vi "Test Program.vi"() -> ()   [LabVIEW 2018, in "VICI M50.lvlib"]
uses:
  VICI M50/VICI M50.lvlib
  Settings Cluster.ctl
  VICI M6 M50 Party Mode.lvlib
panel:
  out "Connection Error":bool
  out "Pump On?":enum16{"Off", "On", "Not Initialized"}(ring)
  in  "stop":bool
  in  "Pause":bool
  in  "speed":dbl
  out "error in (no error) 2":errorcluster
  in  "error in (no error)":errorcluster
  out "VICI Settings 2":T1={"VISA resource name"="", "Simulated?"=TRUE, "Pump Letter"="", "Reverse?"=FALSE}
  in  "VICI Settings":T1={"VISA resource name"="", "Simulated?"=TRUE, "Pump Letter"="", "Reverse?"=FALSE}
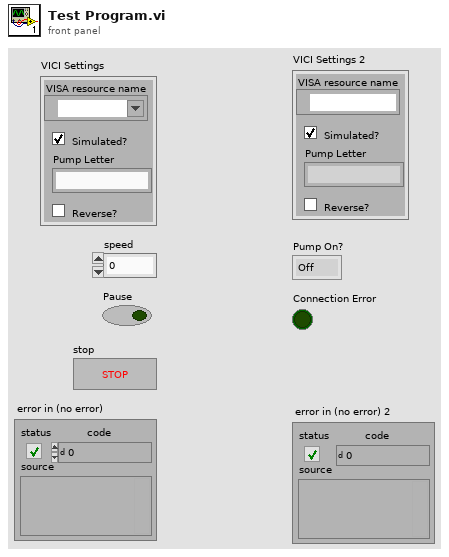
[diagram p1: front panel]
types:
  T1 = typedef "VICI M6 M50 Party Mode.lvlib/Settings Cluster.ctl" = cluster{"VISA resource name":refnum<visa-resource-name>, "Simulated?":bool, "Pump Letter":string, "Reverse?":bool}
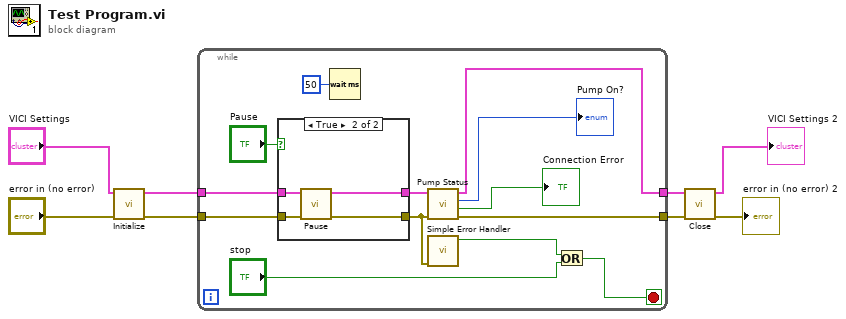
[diagram p0: block diagram]
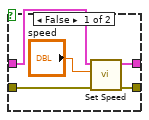
[diagram p2: hidden frame]
diagram:
  n1 = call "Initialize.vi"("error in (no error)"="error in (no error)", "VICI Settings"="VICI Settings") -> ("error out"=w1:errorcluster, "VICI Settings"=w2:T1)  [unwired: 6 in, 2 out]
  n2 = while {
    tunnel: [w21] -> w4
    tunnel: [w20] -> w3
    tunnel: w2 -> [w18]
    tunnel: w1 -> [w17]
    stop <- w13 stop-if-true
    n3 = case shown="True" "Pause" {
      tunnel: [w23 w30] -> w19
      tunnel: [w24 w29] -> w10
      tunnel: w18 -> [w26 w28]
      tunnel: w17 -> [w25 w27]
      frame False {
        n4 = call "Set Speed.vi"("error in (no error)"=w25, "speed"="speed", "VICI Settings In"=w26) -> ("error out"=w24:errorcluster, "VICI Settings Out"=w23:T1)  [unwired: 6 in, 1 out]
      }
      frame True {
        n5 = call "Pause.vi"("error in (no error)"=w27, "VICI Settings In"=w28) -> ("error out"=w29:errorcluster, "VICI Settings Out"=w30:T1)  [unwired: 7 in, 1 out]
      }
    }
    n6 = Wait (ms)(milliseconds to wait=u32 50) -> ()  [unwired: 1 out]
    n7 = call "Pump Status.vi"("error in (no error)"=w10, "VICI Settings In"=w19) -> ("error out"=w20:errorcluster, "Connection Error"=→"Connection Error":bool, "Pump On?"=→"Pump On?":enum16{"Off", "On", "Not Initialized"}, "VICI Settings Out"=w21:T1)  [unwired: 6 in]
    n8 = call <vilib>:"Simple Error Handler.vi"("error in (no error)"=w10) -> ("error?"=w12:bool)  [unwired: 4 in, 4 out]
    n9 = Or(x=w12, y="stop") -> (x .or. y?=w13:bool)
  }
  n10 = call "Close.vi"("error in (no error)"=w3, "VICI Settings"=w4) -> ("error out"=→"error in (no error) 2":errorcluster, "VICI Settings"=→"VICI Settings 2":T1)  [unwired: 7 in, 1 out]
